vi "setClaseReceta.vi"(8 "error in":errorcluster, 10 "dataToSet":T1, 11 "claseReceta in":refnum<class "claseReceta.lvclass">) -> (0 "error out":errorcluster, 3 "claseReceta out":refnum<class "claseReceta.lvclass">)   [LabVIEW 2014, in "claseReceta.lvclass"]
uses:
  claseReceta.lvclass
  claseReceta.lvclass/claseReceta.ctl
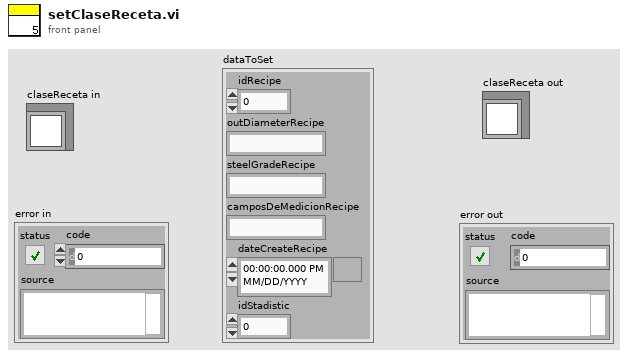
[diagram p1: front panel]
types:
  T1 = cluster{"idRecipe":dbl, "outDiameterRecipe":string, "steelGradeRecipe":string, "camposDeMedicionRecipe":string, "dateCreateRecipe":timestamp, "idStadistic":dbl}
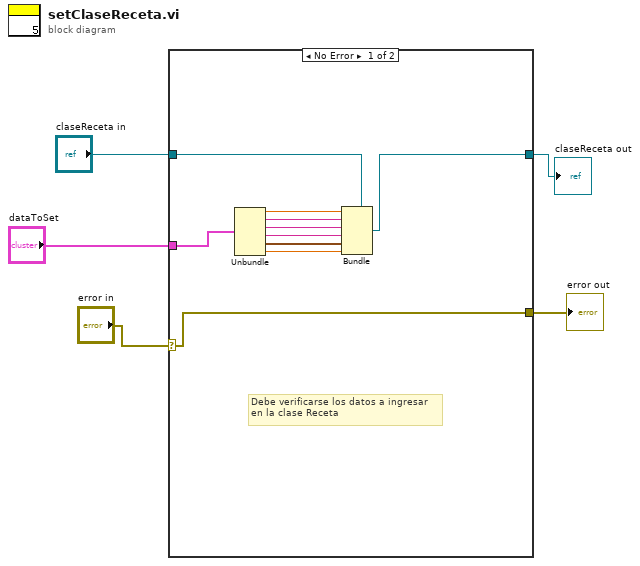
[diagram p0: block diagram]
diagram:
  n1 = case shown="No Error" "error in" {
    selector: "error in" -> [w15 w17]
    tunnel: [w15 w17] -> w4
    tunnel: "claseReceta in" -> [w14 w16]
    tunnel: [w13 w16] -> w2
    tunnel: "dataToSet" -> [w12 _]
    frame No Error {
      # "Debe verificarse los datos a ingresar \nen la clase Receta"
      n2 = Unbundle(w12) -> ("idRecipe"=w11:dbl, "outDiameterRecipe"=w10:string, "steelGradeRecipe"=w9:string, "camposDeMedicionRecipe"=w8:string, "dateCreateRecipe"=w7:timestamp, "idStadistic"=w6:dbl)
      n3 = Bundle(cluster=w14, w11, w10, w9, w8, w7, w6) -> (w13:refnum<class "claseReceta.lvclass">)
    }
    frame Error {
    }
  }
  "claseReceta out" <- w2
  "error out" <- w4
